vi "Better MessageBox.vi"(0 "Title":string, 2 "Parent VI":refnum<vi>, 5 "Message":string, 7 "Icon Style":enum16{"Warning", "Error", "Info", "Question"}(ring), 9 "Text.Font:Size":u32, 11 "Text.Justification":enum16{"Left", "Center", "Right"}(ring)=enum."Center", 12 "Yes text":string="OK", 13 "No text":string="Cancel") -> (8 "Yes response":bool)   [LabVIEW 2020]
panel:
  in  "Cancel":bool
  out "String":string
  out "Frame":string
  in  "OK":bool
  out "Icon":u16(ring)
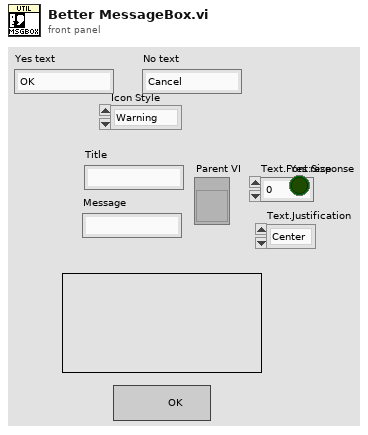
[diagram p1: front panel]
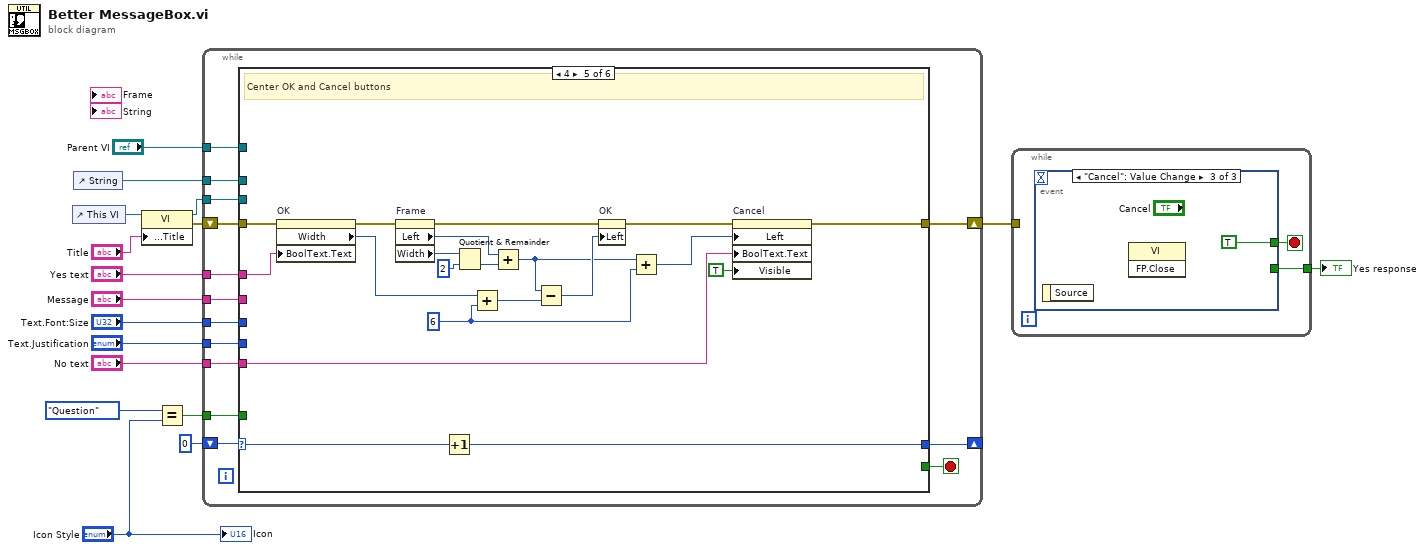
[diagram p0: block diagram]
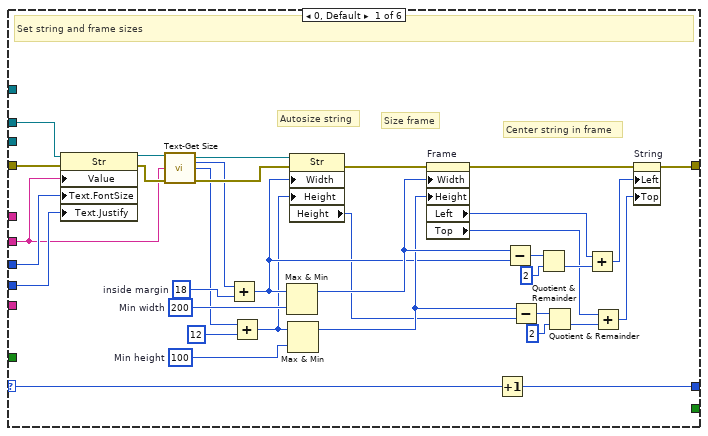
[diagram p2: hidden frame]
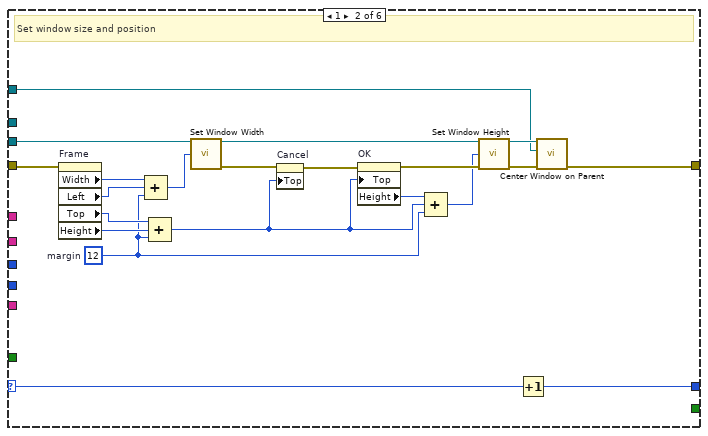
[diagram p3: hidden frame]
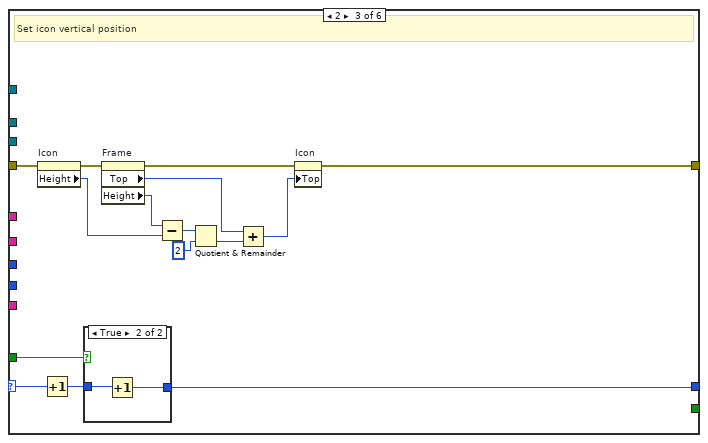
[diagram p4: hidden frame]
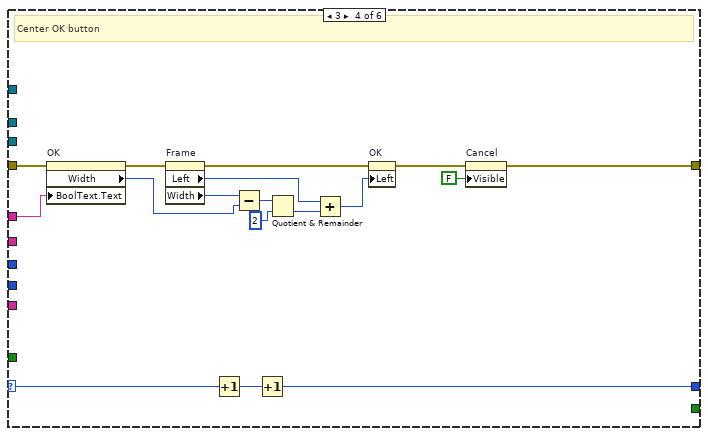
[diagram p6: hidden frame]
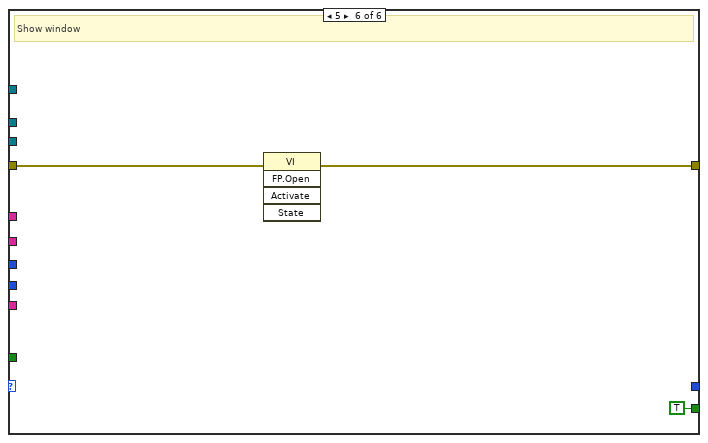
[diagram p7: hidden frame]
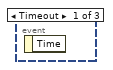
[diagram p8: hidden frame]
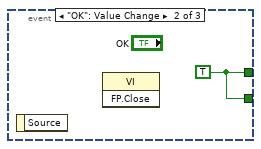
[diagram p9: hidden frame]
diagram:
  n1 = control-ref of="This VI"() -> (w17:refnum<vi>)
  n2 = control-ref of="String"() -> (w12:refnum<vi>)
  n3 = property class="VI"(reference=w17, "Front Panel.Title"="Title") -> (reference out=w9:refnum<vi>, error out=w10:errorcluster)  [unwired: 1 in]
  n4 = Equal?(x=enum16{"Warning", "Error", "Info", "Question"}."Question", y="Icon Style") -> (x = y?=w4:bool)
  n5 = while {
    tunnel: "Text.Font:Size" -> [w30]
    tunnel: "Text.Justification" -> [w29]
    tunnel: w12 -> [w28]
    tunnel: "Message" -> [w27]
    shift-right: [w31] -> w15
    shift-left: w10 -> [w26]
    tunnel: w9 -> [w25]
    tunnel: "Parent VI" -> [w24]
    shift-right: [w22] -> _
    shift-left: 0 -> [w23]
    tunnel: w4 -> [w21]
    tunnel: "Yes text" -> [w19]
    tunnel: "No text" -> [w18]
    stop <- w20 stop-if-true
    n6 = case shown="4" w23 {
      selector: w23 -> [w35 w68 w91 w122 w142 _]
      tunnel: [w36 w86 w92 w107 w134 w144] -> w31
      tunnel: w30 -> [w66 _ _ _ _ _]
      tunnel: w29 -> [w65 _ _ _ _ _]
      tunnel: w28 -> [w64 _ _ _ _ _]
      tunnel: w27 -> [w61 _ _ _ _ _]
      tunnel: w26 -> [w37 w85 w95 w119 w140 w145]
      tunnel: w25 -> [_ w80 _ _ _ _]
      tunnel: w24 -> [_ w69 _ _ _ _]
      tunnel: [w34 w67 w88 w120 w141 _] -> w22
      tunnel: w21 -> [_ _ w89 _ _ _]
      tunnel: [_ _ _ _ _ TRUE] -> w20
      tunnel: w19 -> [_ _ _ w109 w136 _]
      tunnel: w18 -> [_ _ _ _ w129 _]
      frame 0, Default {
        w57 = 18  # inside margin
        w54 = u32 100  # Min height
        w55 = u32 200  # Min width
        # "Size frame"
        # "Autosize string"
        # "Center string in frame"
        # "Set string and frame sizes"
        n7 = property on="Property Node" class="Str"(reference=w64, error in=w37, "Value"=w61, "Text.FontSize"=w66, "Text.Justify"=w65) -> (reference out=w62:refnum<vi>, error out=w63:errorcluster)
        n8 = call "Text-Get Size.vi"("String"=w62, "Text"=w61, "error in (no error)"=w63) -> ("reference out"=w60:refnum<vi>, "width"=w58:i16, "height"=w41:i16, "error out"=w59:errorcluster)  [unwired: 9 in]
        n9 = Add(x=w58, y=w57) -> (x+y=w43:i32)
        n10 = Add(x=w41, y=i16 12) -> (x+y=w33:i16)
        n11 = Max & Min(x=w43, y=w55) -> (max(x,y)=w52:u32)  [unwired: 1 out]
        n12 = Max & Min(x=w33, y=w54) -> (max(x,y)=w44:u32)  [unwired: 1 out]
        n13 = property class="Str"(reference=w60, error in=w59, "Width"=w43, "Height"=w33) -> (error out=w56:errorcluster, "Height"=w40:u32)  [unwired: 1 out]
        n14 = property on="Frame" class="Str"(error in=w56, "Width"=w52, "Height"=w44) -> (error out=w53:errorcluster, "Left"=w38:i32, "Top"=w39:i32)  [unwired: 1 in, 1 out]
        n15 = Increment(x=w35) -> (x+1=w34:i32)
        n16 = Subtract(x=w52, y=w43) -> (x-y=w51:u32)
        n17 = Subtract(x=w44, y=w40) -> (x-y=w47:u32)
        n18 = Quotient & Remainder(x=w51, y=2) -> (floor(x/y)=w49:u32)  [unwired: 1 out]
        n19 = Quotient & Remainder(x=w47, y=2) -> (floor(x/y)=w45:u32)  [unwired: 1 out]
        n20 = Add(x=w38, y=w49) -> (x+y=w48:u32)
        n21 = Add(x=w39, y=w45) -> (x+y=w42:u32)
        n22 = property on="String" class="Str"(error in=w53, "Left"=w48, "Top"=w42) -> (error out=w36:errorcluster)  [unwired: 1 in, 1 out]
      }
      frame 1 {
        w78 = u32 12  # margin
        # "Set window size and position"
        n23 = property on="Frame" class="Str"(error in=w85) -> ("Width"=w84:u32, "Left"=w83:i32, "Top"=w82:i32, "Height"=w81:u32)  [unwired: 1 in, 2 out]
        n24 = Compound Arithmetic op=ADD(w84, w83, w78) -> (w87:u32)
        n25 = Compound Arithmetic op=ADD(w82, w81, w78) -> (w76:u32)
        n26 = call "Set Window Width.vi"("VI in"=w80, "Width"=w87) -> ("VI out"=w74:refnum<vi>, "error out"=w77:errorcluster)  [unwired: 12 in]
        n27 = property on="Cancel" class="Bool"(error in=w77, "Top"=w76) -> (error out=w75:errorcluster)  [unwired: 1 in, 1 out]
        n28 = property on="OK" class="Bool"(error in=w75, "Top"=w76) -> (error out=w73:errorcluster, "Height"=w79:u32)  [unwired: 1 in, 1 out]
        n29 = Compound Arithmetic op=ADD(w79, w76, w78) -> (w72:u32)
        n30 = call "Set Window Height.vi"("VI in"=w74, "Height"=w72, "error in (no error)"=w73) -> ("VI out"=w71:refnum<vi>, "error out"=w70:errorcluster)  [unwired: 11 in]
        n31 = Increment(x=w68) -> (x+1=w67:i32)
        n32 = call "Center Window on Parent.vi"("error in (no error)"=w70, "Parent VI"=w69, "VI in"=w71) -> ("error out"=w86:errorcluster)  [unwired: 7 in, 1 out]
      }
      frame 2 {
        # "Set icon vertical position"
        n33 = property on="Icon" class="Ring (strict)"(error in=w95) -> (error out=w96:errorcluster, "Height"=w100:u32)  [unwired: 1 in, 1 out]
        n34 = Increment(x=w91) -> (x+1=w90:i32)
        n35 = case shown="True" w89 {
          tunnel: w90 -> [w103 w105]
          tunnel: [w103 w104] -> w88
          frame False {
          }
          frame True {
            n36 = Increment(x=w105) -> (x+1=w104:i32)
          }
        }
        n37 = property on="Frame" class="Str"(error in=w96) -> (error out=w94:errorcluster, "Top"=w98:i32, "Height"=w99:u32)  [unwired: 1 in, 1 out]
        n38 = Subtract(x=w99, y=w100) -> (x-y=w102:u32)
        n39 = Quotient & Remainder(x=w102, y=2) -> (floor(x/y)=w97:u32)  [unwired: 1 out]
        n40 = Add(x=w98, y=w97) -> (x+y=w93:u32)
        n41 = property on="Icon" class="Ring (strict)"(error in=w94, "Top"=w93) -> (error out=w92:errorcluster)  [unwired: 1 in, 1 out]
      }
      frame 3 {
        # "Center OK button"
        n42 = property on="OK" class="Bool"(error in=w119, "BoolText.Text"=w109) -> (error out=w118:errorcluster, "Width"=w112:u32)  [unwired: 1 in, 1 out]
        n43 = property on="Frame" class="Str"(error in=w118) -> (error out=w111:errorcluster, "Left"=w113:i32, "Width"=w114:u32)  [unwired: 1 in, 1 out]
        n44 = Increment(x=w122) -> (x+1=w121:i32)
        n45 = Subtract(x=w114, y=w112) -> (x-y=w117:u32)
        n46 = Increment(x=w121) -> (x+1=w120:i32)
        n47 = Quotient & Remainder(x=w117, y=2) -> (floor(x/y)=w115:u32)  [unwired: 1 out]
        n48 = Add(x=w113, y=w115) -> (x+y=w110:u32)
        n49 = property on="OK" class="Bool"(error in=w111, "Left"=w110) -> (error out=w108:errorcluster)  [unwired: 1 in, 1 out]
        n50 = property on="Cancel" class="Bool"(error in=w108, "Visible"=FALSE) -> (error out=w107:errorcluster)  [unwired: 1 in, 1 out]
      }
      frame 4 {
        w127 = u32 6 ("y")
        # "Center OK and Cancel buttons"
        n51 = property on="OK" class="Bool"(error in=w140, "BoolText.Text"=w136) -> (error out=w139:errorcluster, "Width"=w128:u32)  [unwired: 1 in, 1 out]
        n52 = property on="Frame" class="Str"(error in=w139) -> (error out=w137:errorcluster, "Left"=w138:i32, "Width"=w133:u32)  [unwired: 1 in, 1 out]
        n53 = Increment(x=w142) -> (x+1=w141:i32)
        n54 = Quotient & Remainder(x=w133, y=u32 2) -> (floor(x/y)=w131:u32)  [unwired: 1 out]
        n55 = Add(x=w128, y=w127) -> (x+y=w126:u32)
        n56 = Add(x=w138, y=w131) -> (x+y=w124:u32)
        n57 = Subtract(x=w124, y=w126) -> (x-y=w125:u32)
        n58 = property on="OK" class="Bool"(error in=w137, "Left"=w125) -> (error out=w135:errorcluster)  [unwired: 1 in, 1 out]
        n59 = Add(x=w124, y=w127) -> (x+y=w130:u32)
        n60 = property on="Cancel" class="Bool"(error in=w135, "Left"=w130, "BoolText.Text"=w129, "Visible"=TRUE) -> (error out=w134:errorcluster)  [unwired: 1 in, 1 out]
      }
      frame 5 {
        # "Show window"
        n61 = invoke class="VI" method="FP.Open"(error in=w145) -> (error out=w144:errorcluster)  [unwired: 4 in, 4 out]
      }
    }
  }
  n62 = while {
    tunnel: w15 -> [_]
    tunnel: [w146] -> w3
    stop <- w147 stop-if-true
    n63 = event shown="[2] \"Cancel\": Value Change" {
      selector: _ -> [_ _ _]
      dyn-events: _ -> [_ _ _]
      timeout: _ -> [_ _ _]
      tunnel: [_ w148 TRUE] -> w147
      tunnel: [_ w148 _] -> w146
      event Timeout {
        n64 = event-data() -> ()  [unwired: 1 in, 1 out]
      }
      event "OK": Value Change {
        w148 = TRUE
        n65 = event-data() -> ()  [unwired: 1 in, 1 out]
        n66 = invoke class="VI" method="FP.Close"() -> ()  [unwired: 3 in, 3 out]
      }
      event "Cancel": Value Change {
        n67 = event-data() -> ()  [unwired: 1 in, 1 out]
        n68 = invoke class="VI" method="FP.Close"() -> ()  [unwired: 3 in, 3 out]
      }
    }
  }
  "Yes response" <- w3
  "Icon" <- "Icon Style"
